vi "Pose3d_Minus.vi"(9 "other Pose3d":T5={"Translation3d"={"X"=0.0, "Y"=0.0, "Z"=0.0}, "Rotation3d"={"Q_quaternion"={"R"=1.0, "V"=[0.0, 0.0, 0.0]}}} {"Translation3d"."Z" format="%14.3f"; "Translation3d"."Y" format="%14.3f"; "Translation3d"."X" format="%14.3f"}, 11 "in Pose3d":T5={"Translation3d"={"X"=0.0, "Y"=0.0, "Z"=0.0}, "Rotation3d"={"Q_quaternion"={"R"=1.0, "V"=[0.0, 0.0, 0.0]}}} {"Translation3d"."Z" format="%14.3f"; "Translation3d"."Y" format="%14.3f"; "Translation3d"."X" format="%14.3f"}) -> (3 "outTransform3d":T1={"TRANSLATION3D"={"X"=0.0, "Y"=0.0, "Z"=0.0}, "ROTATION3D"={"Q_quaternion"={"R"=1.0, "V"=[0.0, 0.0, 0.0]}}, "XF"=FALSE} {"TRANSLATION3D"."Z" format="%14.3f"; "TRANSLATION3D"."Y" format="%14.3f"; "TRANSLATION3D"."X" format="%14.3f"})   [LabVIEW 2019, in "Trajectory_Library.lvlib"]
doc: "Returns the Transform2d that maps the one pose to another.\n\nParameter:\n - IN POSE - Current POSE data structure\n - OTHER POSE - The initial pose of the transformation.\n\nReturns:\n - OUT TRANSFORMATION - The transform that maps the other pose to the current pose."
uses:
  Trajectory_Library.lvlib
  TRANSLATION3D.ctl
  QUATERNION.ctl
  ROTATION3D.ctl
  POSE3D.ctl
  TRANSFORM3D.ctl
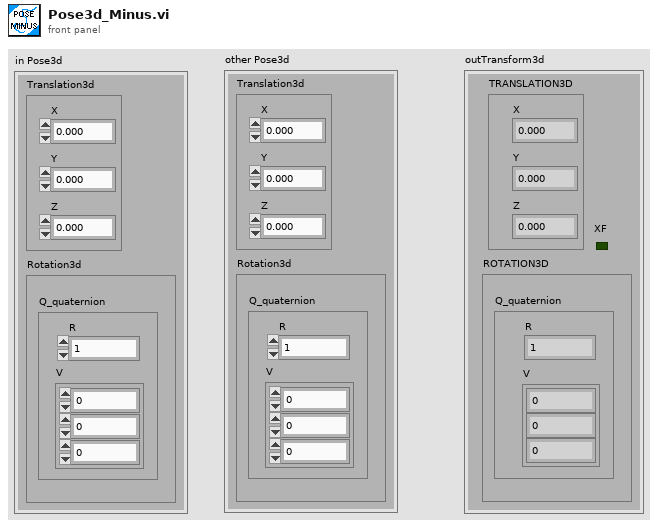
[diagram p1: front panel]
types:
  T1 = typedef "Trajectory_Library.lvlib/TRANSFORM3D.ctl" = cluster{"TRANSLATION3D":T2, "ROTATION3D":T3, "XF":bool}
  T2 = typedef "Trajectory_Library.lvlib/TRANSLATION3D.ctl" = cluster{"X":dbl, "Y":dbl, "Z":dbl}
  T3 = typedef "Trajectory_Library.lvlib/ROTATION3D.ctl" = cluster{"Q_quaternion":T4}
  T4 = typedef "Trajectory_Library.lvlib/QUATERNION.ctl" = cluster{"R":dbl, "V":dbl[]}
  T5 = typedef "Trajectory_Library.lvlib/POSE3D.ctl" = cluster{"Translation3d":T2, "Rotation3d":T3}
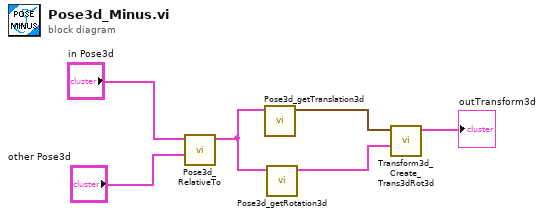
[diagram p0: block diagram]
diagram:
  n1 = call "Pose3d_RelativeTo.vi"("other Pose3d"="other Pose3d", "in Pose3d"="in Pose3d") -> ("out Pose3d"=w4:T5)  [unwired: 9 in]
  n2 = call "Pose3d_getTranslation3d.vi"("in Pose3d"=w4) -> ("out Translation3d"=w3:T2)  [unwired: 10 in]
  n3 = call "Pose3d_getRotation3d.vi"("in Pose3d"=w4) -> ("out Rotation3d"=w2:T3)  [unwired: 10 in]
  n4 = call "Transform3d_Create_Trans3dRot3d.vi"("Rotation3d"=w2, "Translation3d"=w3) -> ("Transform3d"=→"outTransform3d":T1)  [unwired: 9 in]
